vi "WPI_EncoderSetMaxPeriod.vi"(8 "error in (no error)":errorcluster, 10 "MaxPeriod (sec)":dbl=0.05, 11 "EncoderDevRef":T1={"DevStatus"={"status"=FALSE, "code"=0, "source"=""}, "EncoderIndex"=enum."Invalid", "CounterIndex"=enum."Ctr 1", "DistancePerCount"=2.0, "Decoding Type"=enum."4x"}) -> (0 "error out":errorcluster, 3 "EncoderDevRef":T1={"DevStatus"={"status"=FALSE, "code"=0, "source"=""}, "EncoderIndex"=enum."Invalid", "CounterIndex"=enum."Ctr 1", "DistancePerCount"=2.0, "Decoding Type"=enum."4x"})   [LabVIEW 2017]
doc: "Specifies the maximum time between pulses that can elapse before the CompactRIO device considers the encoder to be stopped. Use the Get VI to determine whether the encoder is stopped.\n\nThis software is licensed. Open the labview\\readme\\WPI Robotics Library Open Source License.txt file for more information."
uses:
  <vilib>/Rock Robotics/WPI/Encoder/WPI_EncoderDevRef.ctl
  <vilib>/Rock Robotics/SystemInterfaces/Encoder/FPGA_EncoderIdx.ctl
  <vilib>/Rock Robotics/SystemInterfaces/Counter/FPGA_CounterCtrSystemIndex.ctl
  <vilib>/Rock Robotics/WPI/Encoder/WPI_EncoderType.ctl
  <vilib>/Rock Robotics/SystemInterfaces/Encoder/FPGA_EncoderOpen WO Configuration.vi
  <vilib>/Rock Robotics/SystemInterfaces/Counter/FPGA_CounterERRInvalidResource.vi
  <vilib>/Rock Robotics/SystemInterfaces/Encoder/FPGA_EncoderERRInvalidResource.vi
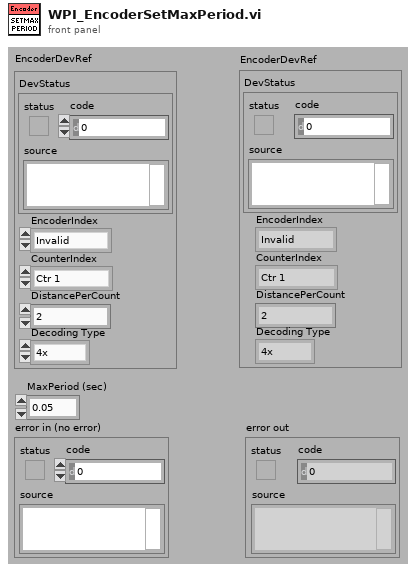
[diagram p1: front panel]
types:
  T1 = typedef "WPI_EncoderDevRef.ctl" = cluster{"DevStatus":errorcluster, "EncoderIndex":T2, "CounterIndex":T3, "DistancePerCount":dbl, "Decoding Type":T4}
  T2 = typedef "FPGA_EncoderIdx.ctl" = enum8{"Enc 0", "Enc 1", "Enc 2", "Enc 3", "Enc 4", "Enc 5", "Enc 6", "Enc 7", "Invalid"}
  T3 = typedef "FPGA_CounterCtrSystemIndex.ctl" = enum8{"Ctr 0", "Ctr 1", "Ctr 2", "Ctr 3", "Ctr 4", "Ctr 5", "Ctr 6", "Ctr 7", "Invalid"}
  T4 = typedef "WPI_EncoderType.ctl" = enum16{"1x", "2x", "4x"}
  T5 = typedef "FPGA_CounterCtrDevRef.ctl" = cluster{"DevStatus":errorcluster, "CntIndex":T3}
  T6 = typedef "FPGA_EncoderDevRef.ctl" = cluster{"EncoderIndex":T2, "DevStatus":errorcluster}
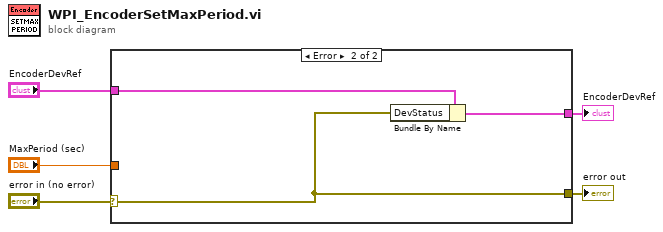
[diagram p0: block diagram]
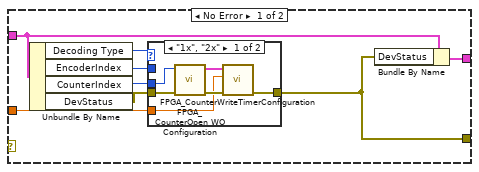
[diagram p2: hidden frame]
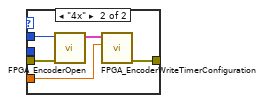
[diagram p3: hidden frame]
diagram:
  n1 = case shown="Error" "error in (no error)" {
    selector: "error in (no error)" -> [_ w25]
    tunnel: "MaxPeriod (sec)" -> [w10 _]
    tunnel: "EncoderDevRef" -> [w8 w27]
    tunnel: [w13 w26] -> w4
    tunnel: [w6 w25] -> w2
    frame No Error {
      n2 = Unbundle By Name(w8) -> ("Decoding Type"=w9:T4, "EncoderIndex"=w11:T2, "CounterIndex"=w7:T3, "DevStatus"=w12:errorcluster)
      n3 = case shown="\"1x\", \"2x\"" w9 {
        tunnel: w12 -> [w18 w24]
        tunnel: w11 -> [_ w23]
        tunnel: w10 -> [w14 w21]
        tunnel: [w19 w20] -> w6
        tunnel: w7 -> [w17 _]
        frame "1x", "2x" {
          n4 = call <vilib>:"FPGA_CounterOpen WO Configuration.vi"("error in"=w18, "CntIndex"=w17) -> ("error out"=w16:errorcluster, "Ctr Ref"=w15:T5)  [unwired: 1 in, 7 out]
          n5 = call <vilib>:"FPGA_CounterWriteTimerConfiguration.vi"("error in (no error)"=w16, "StallPeriod (s)"=w14, "Ctr Ref in"=w15) -> ("error out"=w19:errorcluster)  [unwired: 2 in, 6 out]
        }
        frame "4x" {
          n6 = call-poly <vilib>:"FPGA_EncoderOpen.vi"("DeviceStatus"=w24, "EncoderIndex"=w23) -> ("Encoder Reference"=w22:T6)  [unwired: 1 in, 8 out]
          n7 = call <vilib>:"FPGA_EncoderWriteTimerConfiguration.vi"("StallPeriod (sec)"=w21, "EncoderDevRef"=w22) -> ("error out"=w20:errorcluster)  [unwired: 2 in, 7 out]
        }
      }
      n8 = Bundle By Name(cluster=w8, "DevStatus"=w6) -> (w13:T1)
    }
    frame Error {
      n9 = Bundle By Name(cluster=w27, "DevStatus"=w25) -> (w26:T1)
    }
  }
  "EncoderDevRef" <- w4
  "error out" <- w2
